vi "Fixed_Point.vi"() -> ()   [LabVIEW 2014]
panel:
  out "e/f":fxp<+/-,33,17>
  out "e*f":fxp<+/-,32,24> format="%#_10g"
  in  "e":fxp<+/-,16,12> format="%#_10g"
  in  "f":fxp<+/-,16,12> format="%#_10g"
  out "c-d":fxp<+/-,17,13>
  in  "c":fxp<+/-,16,12> format="%#_10g"
  in  "d":fxp<+/-,16,12> format="%#_10g"
  out "a-b":fxp<+/-,17,13> format="%#_10g"
  out "a+b":fxp<+,17,13> format="%#.10f"
  in  "b":fxp<+,16,12> format="%#_10g"
  in  "a":fxp<+,16,12> format="%#_10g"
  # "Addition\n<+,A,B> + <+,A,B> = <+,A+1,B+1>\n<±,A,B> + <±,A,B> = <±,A+1,B+1>\n\nSubtraction\n<+,A,B> - <+,A,B> = <±,A+1,B+1>\n<±,A,B> - <±,A,B> = <±,A+1,B+1>\n\nMultiply\n<+,A,B> * <+,C,D> = <+A+C,B+D>\n<±,A,B> * <+,C,D> = <±A+C,B+D>\n\nDivision\n<±,A,B> / <±,C,D> = <±,A+C+1,B+C–D+1>\n<+,A,B> /<+,C,D> = <+,A+C, B+C–D>"
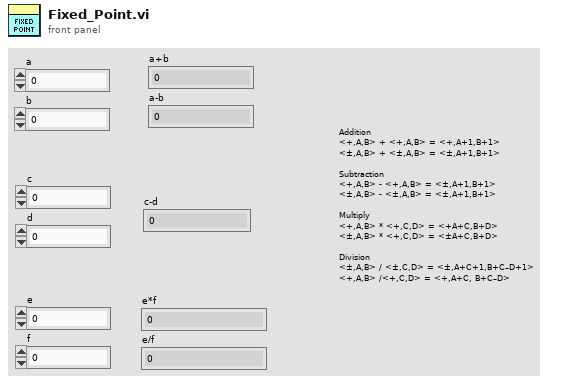
[diagram p1: front panel]
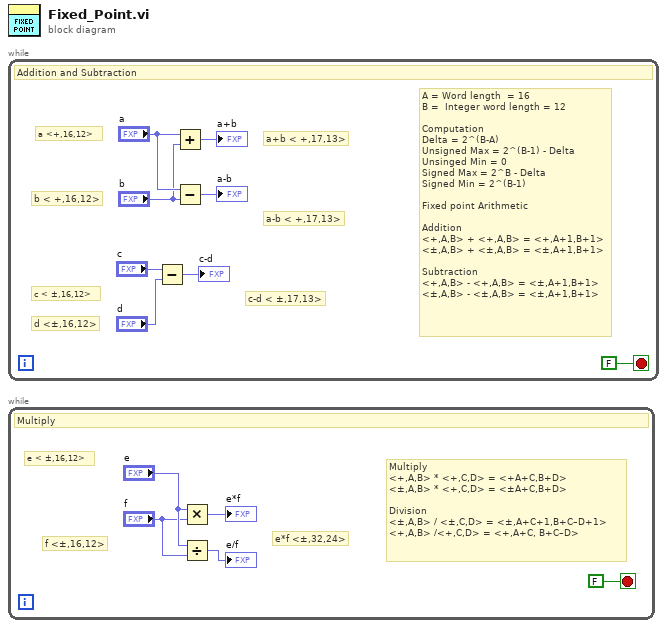
[diagram p0: block diagram]
diagram:
  n1 = while {
    stop <- FALSE stop-if-true
    # "A = Word length  = 16\nB =  Integer word length = 12\n\nComputation\nDelta = 2^(B-A)\nUnsigned Max = 2^(B-1) - Delta\nUnsinged Min = 0\nSigned Max = 2^B - Delta\nSigned Min = 2^(B-1)\n\nFixed point Arithmetic\n\nAddition\n<+,A,B> + <+,A,B> = <+,A+1,B+1>\n<±,A,B> + <±,A,B> = <±,A+1,B+1>\n\nSubtraction\n<+,A,B> - <+,A,B> = <±,A+1,B+1>\n<±,A,B> - <±,A,B> = <±,A+1,B+1>"
    # "c-d < ±,17,13>"
    # "a-b < +,17,13>"
    # "a+b < +,17,13>"
    # "d <±,16,12>"
    # "c < ±,16,12>"
    # "b < +,16,12>"
    # "a <+,16,12>"
    # "Addition and Subtraction"
    n2 = Subtract(x="c", y="d") -> (x-y=→"c-d":fxp<+/-,17,13>)
    n3 = Add(x="a", y="b") -> (x+y=→"a+b":fxp<+,17,13>)
    n4 = Subtract(x="a", y="b") -> (x-y=→"a-b":fxp<+/-,17,13>)
  }
  n5 = while {
    stop <- FALSE stop-if-true
    # "Multiply\n<+,A,B> * <+,C,D> = <+A+C,B+D>\n<±,A,B> * <+,C,D> = <±A+C,B+D>\n\nDivision\n<±,A,B> / <±,C,D> = <±,A+C+1,B+C–D+1>\n<+,A,B> /<+,C,D> = <+,A+C, B+C–D>"
    # "e*f <±,32,24>"
    # "f <±,16,12>"
    # "e < ±,16,12>"
    # "Multiply"
    n6 = Multiply(x="e", y="f") -> (x*y=→"e*f":fxp<+/-,32,24>)
    n7 = Divide(x="e", y="f") -> (x/y=→"e/f":fxp<+/-,33,17>)
  }
